vi "Check String to Bool.vi"(1 "string of check":string) -> (0 "Boolean":bool)   [LabVIEW 2016, in "DataGrid.lvlib" / "DataTable.lvclass"]
uses:
  <userlib>/LabVIEWdotNetDataGrid/source/DataTable/DataTable.lvclass
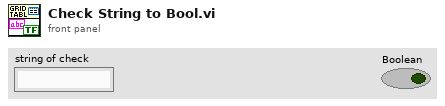
[diagram p1: front panel]
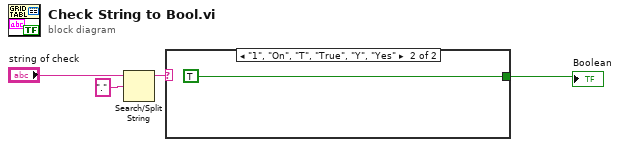
[diagram p0: block diagram]
diagram:
  n1 = Search/Split String(string="string of check", search string/char (-)="." ("regular expression")) -> (substring before match=w1:string)  [unwired: 1 in, 2 out]
  n2 = case shown="\"1\", \"On\", \"T\", \"True\", \"Y\", \"Yes\"" w1 {
    tunnel: [_ TRUE] -> w4
    frame Default {
    }
    frame "1", "On", "T", "True", "Y", "Yes" {
    }
  }
  "Boolean" <- w4
